vi "Info Insert Row to 2D String Array.vi"(6 "source info data":string, 7 "key description":string, 8 "sections in":string[](array[string]), 9 "row index to insert":i32, 10 "row to insert":string[](array[string]), 11 "info data in":string) -> (0 "sections out":string[](array[string]), 3 "info data out":string)   [LabVIEW 2020]
doc: "Addition to infolib: Gets 2D array of strings (if exits in the 'info data in'), inserts one row of strings into it in selected row, writes it back."
uses:
  infolib/Get 2D String.vi
  infolib/2D String.vi
  infolib/infolib.lvlib
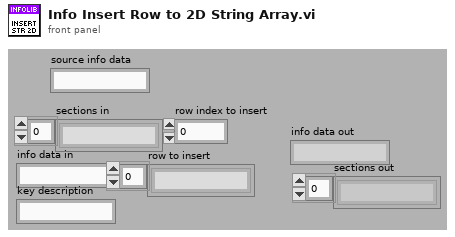
[diagram p1: front panel]
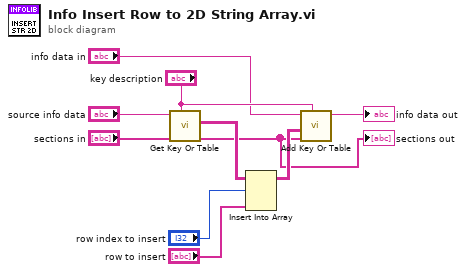
[diagram p0: block diagram]
diagram:
  n1 = call-poly "Get Key Or Table.vi"("key description"="key description", "sections"="sections in", "info data"="source info data") -> ("sections out"=w1:string[], "value"=w10:string[][])  [unwired: 5 in, 2 out]
  "sections out" <- w1
  n2 = Insert Into Array(array=w10, index (row)="row index to insert", new element="row to insert") -> (w7:string[][])  [unwired: 1 in]
  n3 = call-poly "Add Key Or Table.vi"("key description"="key description", "sections"=w1, "string"=w7, "info data"="info data in") -> ("info data out"=→"info data out":string)  [unwired: 6 in, 1 out]
